vi "atomNumberGaussian.vi"(6 "Image bg":sgl[][](array[numeric]) format="%.2f", 8 "error in (no error)":errorcluster, 9 "Image ref":sgl[][](array[numeric]) format="%.2f", 10 "Image object":sgl[][](array[numeric]) format="%.2f", 11 "BECImageProcessor in":refnum<class "BECImageProcessor.lvclass">) -> (0 "error out":errorcluster, 1 "width":dbl, 2 "number":dbl, 3 "BECImageProcessor out":refnum<class "BECImageProcessor.lvclass">)   [LabVIEW 2011, in "Tools.lvlib" / "Imaging.lvlib" / "BECImageProcessor.lvclass"]
uses:
  BECImageProcessor.lvclass
  <vilib>/Analysis/NI_AALBase.lvlib
  <vilib>/Analysis/NI_AALPro.lvlib
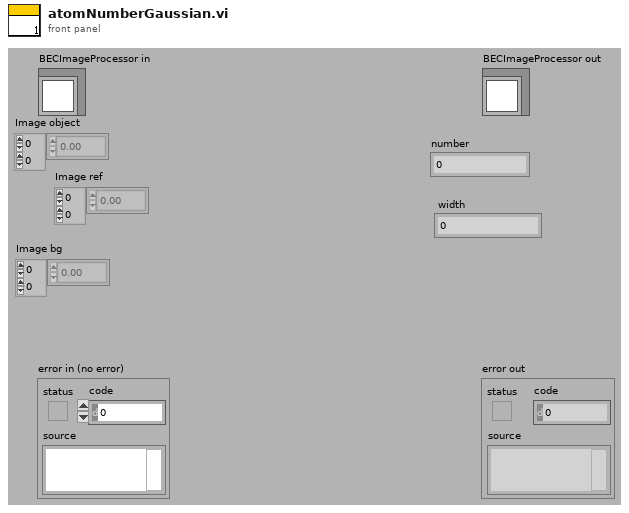
[diagram p1: front panel]
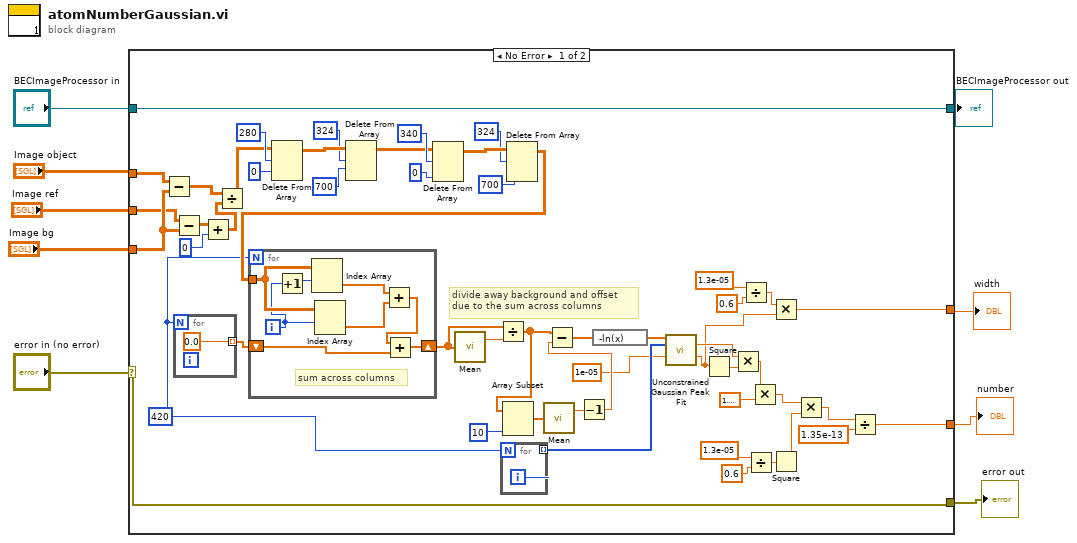
[diagram p0: block diagram]
diagram:
  n1 = case shown="No Error" "error in (no error)" {
    selector: "error in (no error)" -> [w60 w73]
    tunnel: [w60 w73] -> w8
    tunnel: [w61 w72] -> w6
    tunnel: "BECImageProcessor in" -> [w61 w72]
    tunnel: "Image object" -> [w58 _]
    tunnel: "Image ref" -> [w56 _]
    tunnel: "Image bg" -> [w57 _]
    tunnel: [w16 _] -> w2
    tunnel: [w15 _] -> w1
    frame No Error {
      w35 = 420
      # "divide away background and offset\ndue to the sum across columns"
      n2 = Subtract(x=w58, y=w57) -> (x-y=w59:sgl[][])
      n3 = Subtract(x=w56, y=w57) -> (x-y=w13:sgl[][])
      n4 = for {
        N: w35 -> [_]
        tunnel: [0.0] -> w42 mode=indexing
      }
      n5 = Add(x=w13, y=0) -> (x+y=w12:sgl[][])
      n6 = Divide(x=w59, y=w12) -> (x/y=w44:sgl[][])
      n7 = Delete From Array(array=w44, length=280, index (row)=0) -> (array with subset deleted=w53:sgl[][])  [unwired: 1 in, 1 out]
      n8 = Delete From Array(array=w53, length=324, index (row)=700) -> (array with subset deleted=w47:sgl[][])  [unwired: 1 in, 1 out]
      n9 = Delete From Array(array=w47, length=340, index (col)=0) -> (array with subset deleted=w49:sgl[][])  [unwired: 1 in, 1 out]
      n10 = for {
        N: w35 -> [_]
        tunnel: [w62] -> w32 mode=indexing
        i -> [w62]
      }
      n11 = Delete From Array(array=w49, length=324, index (col)=700) -> (array with subset deleted=w43:sgl[][])  [unwired: 1 in, 1 out]
      n12 = for {
        N: w35 -> [_]
        tunnel: w43 -> [w71]
        shift-right: [w66] -> w41
        shift-left: w42 -> [w67]
        i -> [w64]
        # "sum across columns"
        n13 = Increment(x=w64) -> (x+1=w65:i32)
        n14 = Index Array(array=w71, index (row)=w65) -> (element=w70:sgl[])  [unwired: 1 in]
        n15 = Index Array(array=w71, index (row)=w64) -> (element=w69:sgl[])  [unwired: 1 in]
        n16 = Add(x=w70, y=w69) -> (x+y=w68:sgl[])
        n17 = Add(x=w68, y=w67) -> (x+y=w66:dbl[])
      }
      n18 = call <vilib>:"Mean.vi"("X"=w41) -> ("mean"=w10:dbl)  [unwired: 1 out]
      n19 = Divide(x=w41, y=w10) -> (x/y=w37:dbl[])
      n20 = Array Subset(array=w37, length=10) -> (w40:dbl[])  [unwired: 1 in]
      n21 = call <vilib>:"Mean.vi"("X"=w40) -> ("mean"=w39:dbl)  [unwired: 1 out]
      n22 = Decrement(x=w39) -> (x-1=w36:dbl)
      n23 = Subtract(x=w37, y=w36) -> (x-y=w34:dbl[])
      n24 = expression code="-ln(x)"(w34) -> (w33:dbl[])
      n25 = call <vilib>:"Unconstrained Gaussian Peak Fit.vi"("Y"=w33, "X"=w32, "tolerance"=1e-05) -> ("amplitude"=w21:dbl, "standard deviation"=w17:dbl)  [unwired: 7 in, 4 out]
      n26 = Square(x=w17) -> (x^2=w23:dbl)
      n27 = Multiply(x=w21, y=w23) -> (x*y=w22:dbl)
      n28 = Divide(x=1.3e-05, y=0.6) -> (x/y=w18:dbl)
      n29 = Divide(x=1.3e-05, y=0.6) -> (x/y=w26:dbl)
      n30 = Multiply(x=w22, y=1.5707963267948966) -> (x*y=w31:dbl)
      n31 = Multiply(x=w18, y=w17) -> (x*y=w16:dbl)
      n32 = Square(x=w26) -> (x^2=w25:dbl)
      n33 = Multiply(x=w31, y=w25) -> (x*y=w29:dbl)
      n34 = Divide(x=w29, y=1.35e-13) -> (x/y=w15:dbl)
    }
    frame Error {
    }
  }
  "error out" <- w8
  "BECImageProcessor out" <- w6
  "width" <- w2
  "number" <- w1
